vi "Example.vi"() -> ()   [LabVIEW 2024]
uses:
  bitrate.ctl
  message.ctl
  message type.ctl
  ecc register.ctl
  ecc register error code.ctl
  ecc register direction.ctl
  ecc register segment.ctl
  <vilib>/Utility/sysdir.llb/System Directory Type.ctl
  atsj peakcan basic.lvlib
panel:
  out "current log dir":string
  out "current api version":string
  out "results":cluster{"message":T1, "ecc register":T3}[](array[cluster]) {"message"."id" format="%x"; "message"."data" format="%x"}
  out "error":errorcluster
  in  "stop":bool
  in  "bitrate":T7=enum."RATE_1Mbps"
  in  "ip address":string="192.168.2.1"
  # "implemented in api version 4.10.1.968"
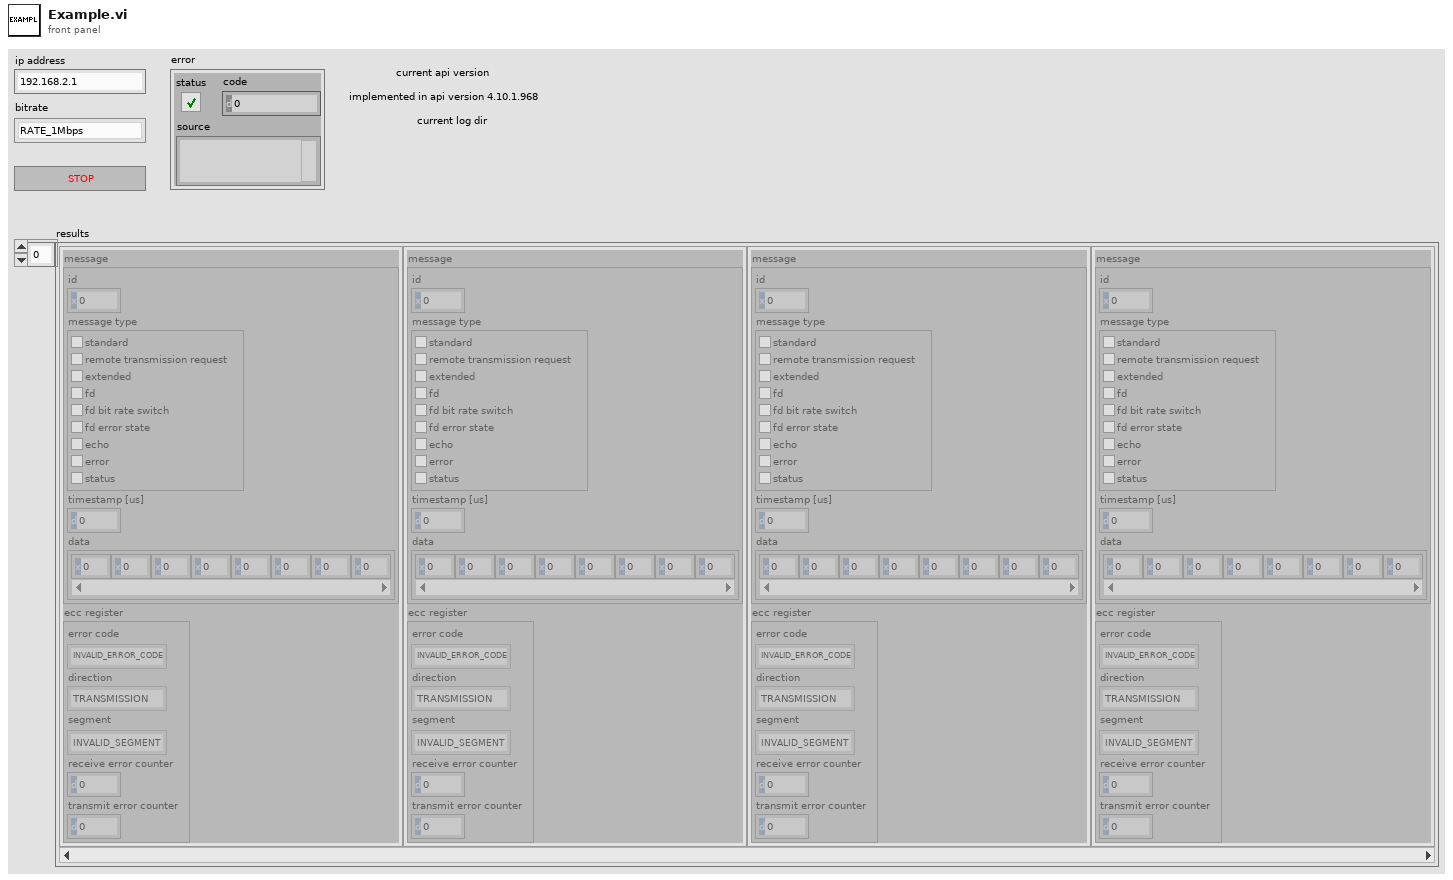
[diagram p1: front panel]
types:
  T1 = typedef "atsj peakcan basic.lvlib/message.ctl" = cluster{"id":u32, "message type":T2, "timestamp [us]":u64, "data":u8[]}
  T2 = typedef "atsj peakcan basic.lvlib/message type.ctl" = cluster{"standard":bool, "remote transmission request ":bool, "extended":bool, "fd":bool, "fd bit rate switch":bool, "fd error state":bool, "echo":bool, "error":bool, "status":bool}
  T3 = typedef "atsj peakcan basic.lvlib/ecc register.ctl" = cluster{"error code":T4, "direction":T5, "segment":T6, "receive error counter":u8, "transmit error counter":u8}
  T4 = typedef "atsj peakcan basic.lvlib/ecc register error code.ctl" = enum8{"INVALID_ERROR_CODE", "COUNTERS_UPDATE", "BIT_ERROR", "FORM_ERROR", "STUFF_ERROR", "OTHER_ERROR"}
  T5 = typedef "atsj peakcan basic.lvlib/ecc register direction.ctl" = enum16{"TRANSMISSION", "RECEPTION"}
  T6 = typedef "atsj peakcan basic.lvlib/ecc register segment.ctl" = enum8{"INVALID_SEGMENT", "ID_28_TO_ID_21", "START_OF_FRAME", "BIT_SRTR", "BIT_IDE", "ID_20_TO_ID_18", "ID_17_TO_ID_13", "CRC_SEQUENCE", "RESERVED_BIT_0", "DATA_FIELD", "DATA_LENGTH_CODE", "BIT_RTR", "RESERVED_BIT_1", "ID_4_TO_ID_0", "ID_12_TO_ID_5", "ACTIVE_ERROR_FLAG", "INTERMISSION", "TOLERATE_DOMINANT_BITS", "ERROR_DELIMITER", "CRC_DELIMITER", "ACKNOWLEDGE_SLOT", "END_OF_FRAME", "ACKNOWLEDGE_LIMITER", "OVERLOAD_FLAG"}
  T7 = typedef "atsj peakcan basic.lvlib/bitrate.ctl" = enum16{"RATE_UNSUPPORTED", "RATE_1Mbps", "RATE_800kbps", "RATE_500kbps", "RATE_250kbps", "RATE_125kbps", "RATE_100kbps", "RATE_95kbps", "RATE_83kbps", "RATE_50kbps", "RATE_47kbps", "RATE_33kbps", "RATE_20kbps", "RATE_10kbps", "RATE_5kbps"}
  T8 = typedef "System Directory Type.ctl" = i32
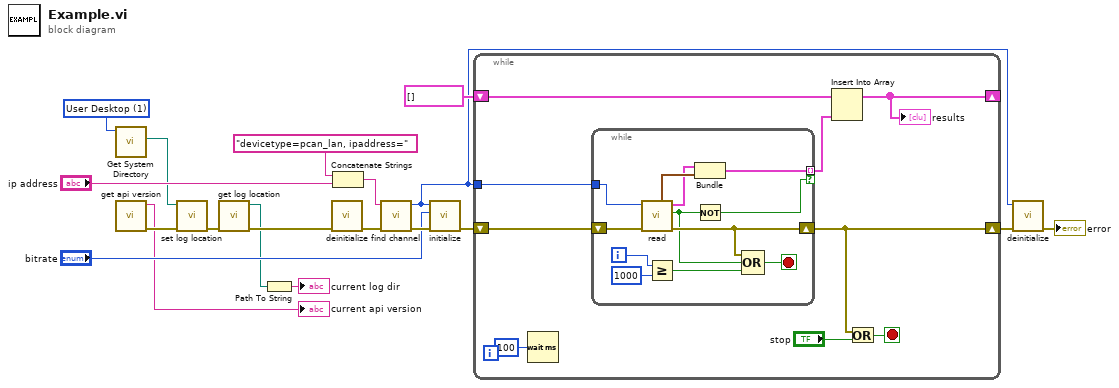
[diagram p0: block diagram]
diagram:
  w3 = T8 1 items=["User Home"=0, "User Desktop"=1, "User Documents"=2, "User Application Data"=3, "User Preferences"=4, "User Temporary"=5, "Public Documents"=6, "Public Application Data"=7, "Public Preferences"=8, "Public Cache"=13, "System Core Libraries"=9, "System Installed Libraries"=10, "Application Files"=11, "Boot Volume Root"=12] ("system directory type")
  n1 = call <vilib>:"Get System Directory.vi"("system directory type"=w3) -> ("system directory"=w4:path)  [unwired: 10 in]
  n2 = call "get api version.vi"() -> ("error out"=w8:errorcluster, "api version"=→"current api version":string)  [unwired: 10 in]
  n3 = call "set log location.vi"("error in (no error)"=w8, "log directory"=w4) -> ("error out"=w7:errorcluster)  [unwired: 9 in]
  n4 = call "get log location.vi"("error in (no error)"=w7) -> ("error out"=w6:errorcluster, "log directory"=w2:path)  [unwired: 9 in]
  n5 = Path To String(path=w2) -> (string=→"current log dir":string)
  n6 = call "deinitialize.vi"("error in (no error)"=w6) -> ("error out"=w19:errorcluster)  [unwired: 10 in]
  n7 = Concatenate Strings("devicetype=pcan_lan, ipaddress=", "ip address") -> (w13:string)
  n8 = call "find channel.vi"("error in (no error)"=w19, "lookup string"=w13) -> ("error out"=w18:errorcluster, "channel"=w9:u16)  [unwired: 8 in]
  n9 = call "initialize.vi"("error in (no error)"=w18, "bitrate"="bitrate", "channel"=w9) -> ("error out"=w17:errorcluster)  [unwired: 8 in]
  n10 = while {
    shift-right: [w25] -> w16
    shift-left: w17 -> [w28]
    tunnel: w9 -> [w26]
    shift-right: [w22] -> _
    shift-left: cluster{"message":T1, "ecc register":T3}[] [] -> [w21]
    stop <- w23 stop-if-true
    n11 = Wait (ms)(milliseconds to wait=u32 100) -> ()  [unwired: 1 out]
    n12 = while {
      shift-right: [w33] -> w25
      shift-left: w28 -> [w40]
      tunnel: w26 -> [w39]
      tunnel: [w36] -> w20 mode=indexing if=w29
      i -> [w35]
      stop <- w31 stop-if-true
      n13 = call "read.vi"("error in (no error)"=w40, "channel"=w39) -> ("error out"=w33:errorcluster, "queue empty?"=w30:bool, "message"=w37:T1, "ecc register"=w38:T3)  [unwired: 6 in]
      n14 = Greater Or Equal?(x=w35, y=1000) -> (x >= y?=w32:bool)
      n15 = Bundle("message"=w37, "ecc register"=w38) -> (w36:cluster{"message":T1, "ecc register":T3})  [unwired: 1 in]
      n16 = Not(x=w30) -> (.not. x?=w29:bool)
      n17 = Compound Arithmetic op=OR(w33, w30, w32) -> (w31:bool)
    }
    n18 = Insert Into Array(array=w21, new element=w20) -> (w22:cluster{"message":T1, "ecc register":T3}[])  [unwired: 1 in]
    "results" <- w22
    n19 = Or(x=w25, y="stop") -> (x .or. y?=w23:bool)
  }
  n20 = call "deinitialize.vi"("error in (no error)"=w16, "channel (0:all)"=w9) -> ("error out"=→"error":errorcluster)  [unwired: 9 in]
